vi "FTW-Actor-Log-Event.vi"(0 "Featherweight Actor":refnum<class "FTW-Actor.lvclass">, 5 "Event Type":string, 7 "Event Data":string, 9 "Source (unwired for call chain)":string="CallChain", 11 "error in":errorcluster) -> (4 "Featherweight Actor out":refnum<class "FTW-Actor.lvclass">, 6 "Serialized Event":string, 15 "error out":errorcluster)   [LabVIEW 2013, in "FTW-Actor.lvclass"]
uses:
  FTW-Actor.lvclass
  FTW-Actor.lvclass/FTW-Actor.ctl
  Logging/FTW-EventLogger-API.lvclass
panel:
  # "Inputs"
  # "Outputs"
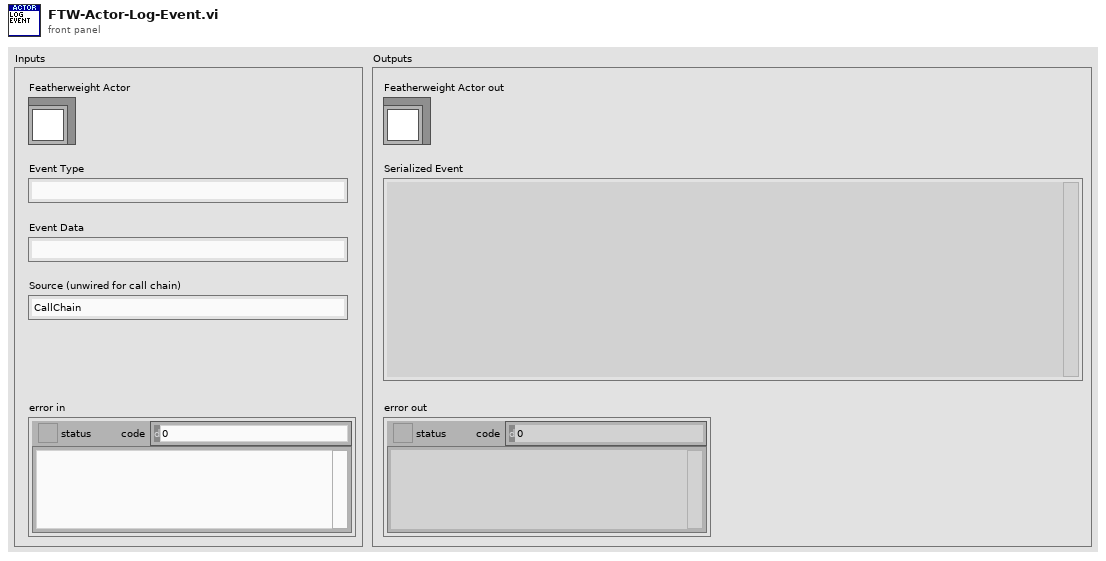
[diagram p1: front panel]
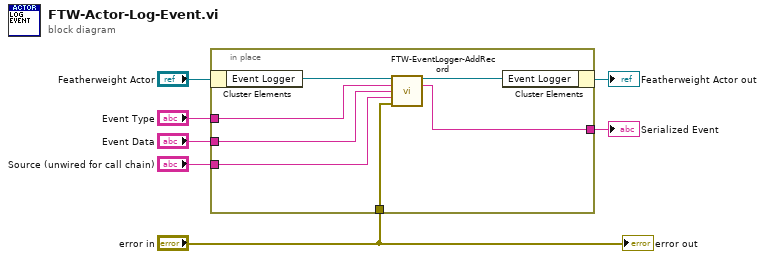
[diagram p0: block diagram]
diagram:
  n1 = in-place {
    in-place-border: "error in" -> [w14]
    in-place-border: [w11] -> w5
    in-place-border: "Event Type" -> [w10]
    in-place-border: "Event Data" -> [w9]
    in-place-border: "Source (unwired for call chain)" -> [w8]
    n2 = in-place-cluster #1("Featherweight Actor") -> ("Event Logger"=w13:refnum<class "FTW-EventLogger-API.lvclass">)
    n3 = call "FTW-EventLogger-AddRecord.vi"("Event Logger"=w13, "Event Type"=w10, "Event Data"=w9, "Source (unwired for call chain)"=w8, "Error to Log"=w14) -> ("Event Logger out"=w12:refnum<class "FTW-EventLogger-API.lvclass">, "Serialized Event"=w11:string)  [unwired: 9 in]
    n4 = in-place-cluster #1("Event Logger"=w12) -> (→"Featherweight Actor out":refnum<class "FTW-Actor.lvclass">)
  }
  "Serialized Event" <- w5
  "error out" <- "error in"
